vi "Interlock View.vi"(11 "Model in":refnum<class "Model.lvclass">) -> ()   [LabVIEW 2016, in "M1M3SupportEUI_Views.lvlib"]
uses:
  M1M3SupportEUI_Views.lvlib
  Model/Model.lvclass
  M1M3 Support Events/M1M3 Support Events.lvclass/M1M3 Support Events.ctl
  M1M3 Support Events/M1M3 Support Events.lvclass
panel:
  out "GIS Heartbeat Lost":string
  out "TMA Motion Stop":string
  out "Air Supply":string
  out "Thermal Equipment":string
  out "HB Output":string
  out "HB Command":string
  out "Aux Power":string
  out "Heartbeat State":string
  out "AnyWarning":string
  out "Interlock Status Time Stamp":timestamp
  out "Interlock Warning Time Stamp":timestamp
  # "Interlock Event Data"
  # "Warnings"
  # "Status"
  # "Heartbeat Commanded State"
  # "Any Warning"
  # "Heartbeat Output State"
  # "Heartbeat State Output Mismatch"
  # "Critical Fault State Output Mismatch"
  # "Thermal Equipment Off"
  # "Air Supply Off"
  # "TMA Motion Stop"
  # "GIS Heartbeat Lost"
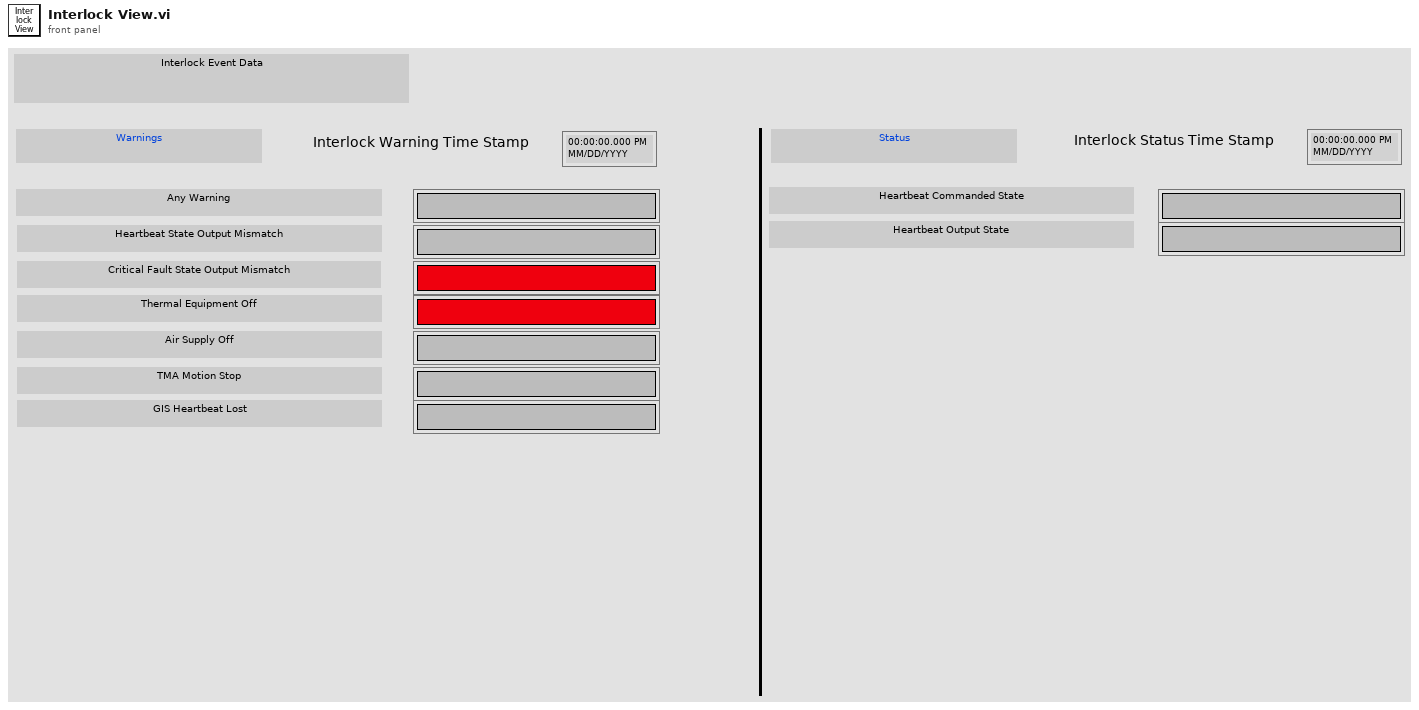
[diagram p1: front panel]
types:
  T1 = typedef "M1M3SupportEUI_TypeDefs.lvlib/M1M3 Support Events.ctl" = cluster{"Inclinometer  Data":refnum<user-event>, "IMS Data":refnum<user-event>, "SAL Connected":refnum<user-event>, "Accelerometer Data":refnum<user-event>, "OuterLoop Data":refnum<user-event>, "ErrorCode Event":refnum<user-event>, "InterlockStatus Event":refnum<user-event>, "InterlockWarning Event":refnum<user-event>, "Gyro Data":refnum<user-event>, "HP Actuator Info Event":refnum<user-event>, " FA Info Event":refnum<user-event>, "HP Monitor Info Event":refnum<user-event>, "FA Data":refnum<user-event>, "HP Actuator data":refnum<user-event>, "HP Monitor data":refnum<user-event>, "Air Supply Status Event":refnum<user-event>, "Air Supply Warning Event":refnum<user-event>, "Power Data":refnum<user-event>, "PID Data":refnum<user-event>, "PID Info Event":refnum<user-event>, "Power Status Event":refnum<user-event>, "Power Supply Status Event":refnum<user-event>, "Power Warning Event":refnum<user-event>, "Summary State Event":refnum<user-event>, "Detailed State Event":refnum<user-event>, "FA Force Warning Event":refnum<user-event>, "FA Warning Event":refnum<user-event>, "FA State Event":refnum<user-event>, "Applied AberrationForces Event":refnum<user-event>, "Applied Acceleration Forcces Event":refnum<user-event>, "Applied Azimuth Forces Event":refnum<user-event>, "Applied Active Optic Forces Event":refnum<user-event>, "Applied Balance Forces Event":refnum<user-event>, "Applied Cylinder Forces Event":refnum<user-event>, "Applied Elevation Forces Event":refnum<user-event>, "Applied Forces Event":refnum<user-event>, "Applied Offset Forces Event":refnum<user-event>, "Applied Static Forces Event":refnum<user-event>, "Applied Thermal Forces Event":refnum<user-event>, "Applied Velocity Forces Event":refnum<user-event>, "Rejected Aberration Force Event":refnum<user-event>, "Rejected Acceleration Forces Event":refnum<user-event>, "Rejected Active Optic Forces Event":refnum<user-event>, "Rejected Azimuth Forces Event":refnum<user-event>, "Rejected Balance Forces Event":refnum<user-event>, "Rejected Cylinder Forces Event":refnum<user-event>, "Rejected Elevation Forces Event":refnum<user-event>, "Rejected Forces Event":refnum<user-event>, "Rejected Offset Forces Event":refnum<user-event>, "Rejected Static Forces Event":refnum<user-event>, "Rejected Thermal Forces Event":refnum<user-event>, "Rejected Velocity Forces Event":refnum<user-event>, "Command Rejection Event":refnum<user-event>, "Setting Verions Event":refnum<user-event>, "Settings Applied Event":refnum<user-event>}
  T2 = enum16{"", "DetailedState_DetailedStates_DisabledState", "DetailedState_DetailedStates_EnabledState", "DetailedState_DetailedStates_FaultState", "DetailedState_DetailedStates_OfflineState", "DetailedState_DetailedStates_StandbyState", "DetailedState_DetailedStates_ParkedState", "DetailedState_DetailedStates_RaisingState", "DetailedState_DetailedStates_ActiveState", "DetailedState_DetailedStates_LoweringState", "DetailedState_DetailedStates_EngineeringState", "DetailedState_DetailedStates_ParkedEngineeringState", "DetailedState_DetailedStates_RaisingEngineeringState", "DetailedState_DetailedStates_ActiveEngineeringState", "DetailedState_DetailedStates_LoweringEngineeringState", "DetailedState_DetailedStates_LoweringFaultState", "DetailedState_DetailedStates_ProfileHardpointCorrectionState"}
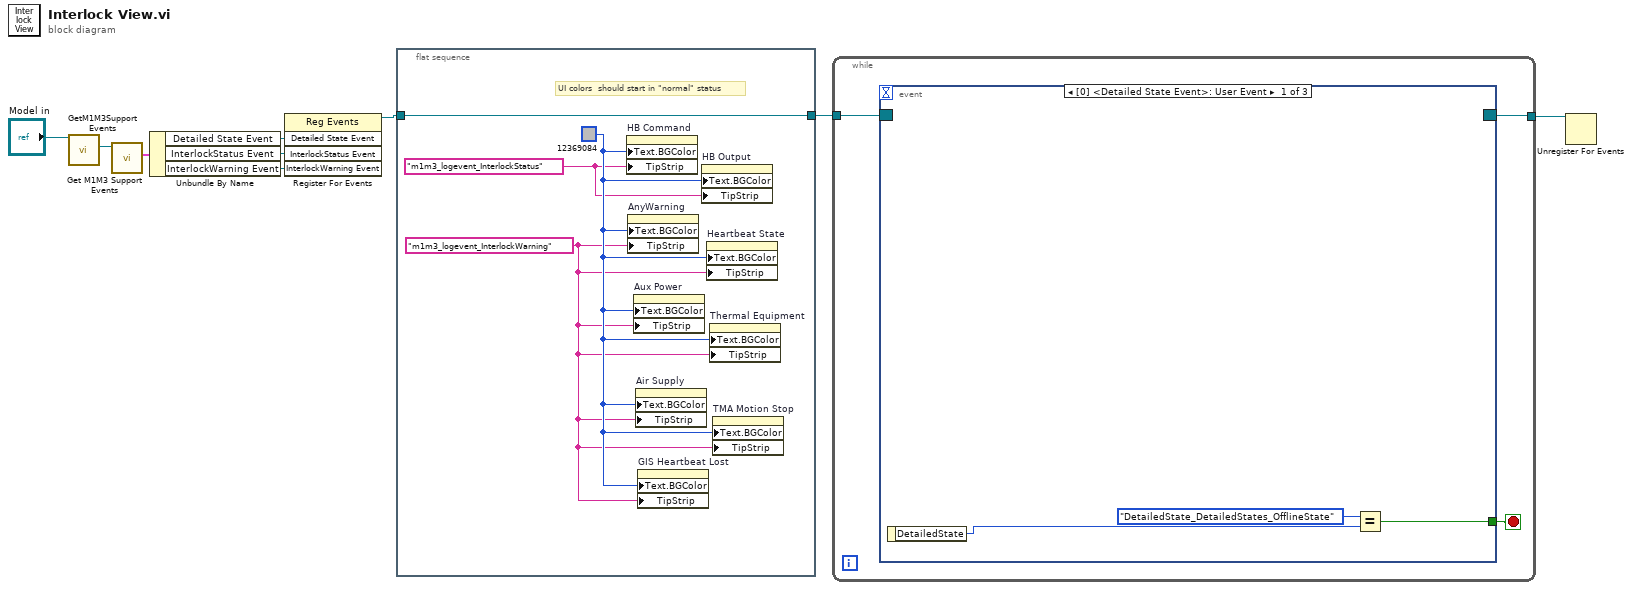
[diagram p0: block diagram]
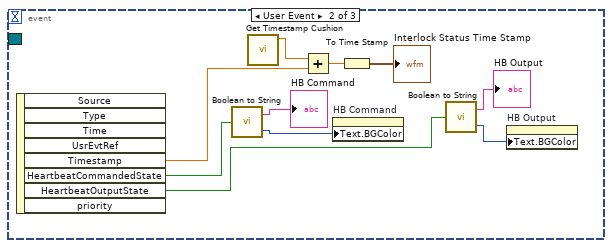
[diagram p2: hidden frame]
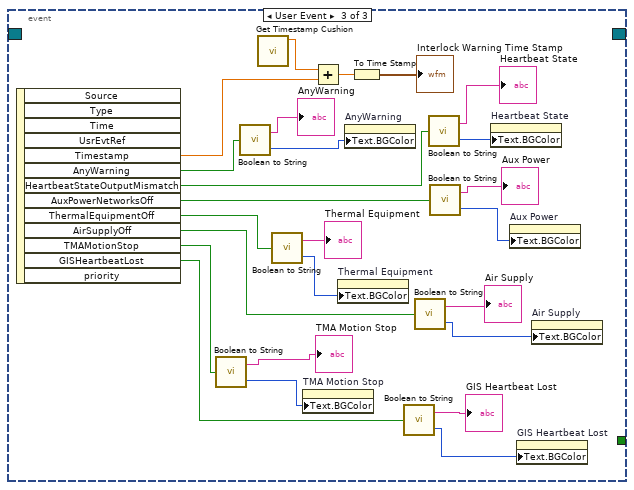
[diagram p3: hidden frame]
diagram:
  n1 = call "GetM1M3SupportEvents.vi"("Model in"="Model in") -> ("M1M3 Support Events out"=w5:refnum<class "M1M3 Support Events.lvclass">)  [unwired: 8 in, 2 out]
  n2 = call "Get M1M3 Support Events.vi"("M1M3 Support Events in"=w5) -> ("M1M3 Support Events"=w6:T1)  [unwired: 9 in, 1 out]
  n3 = Unbundle By Name(w6) -> ("Detailed State Event"=w7:refnum<user-event>, "InterlockStatus Event"=w8:refnum<user-event>, "InterlockWarning Event"=w9:refnum<user-event>)
  n4 = register-events(w7, w8, w9) -> (reference out=w2:refnum<event-registration>)  [unwired: 2 in, 1 out]
  n5 = flat-sequence {
    tunnel: w2 -> [w13]
    tunnel: [w13] -> w1
    frame #0 {
      w10 = "m1m3_logevent_InterlockWarning" ("Tip Strip")
      w11 = "m1m3_logevent_InterlockStatus" ("Tip Strip")
      w12 = u32 12369084
      # "UI colors  should start in \"normal\" status"
      n6 = property on="HB Command" class="Str"("Text.BGColor"=w12, "TipStrip"=w11) -> ()  [unwired: 2 in, 2 out]
      n7 = property on="AnyWarning" class="Str"("Text.BGColor"=w12, "TipStrip"=w10) -> ()  [unwired: 2 in, 2 out]
      n8 = property on="Aux Power" class="Str"("Text.BGColor"=w12, "TipStrip"=w10) -> ()  [unwired: 2 in, 2 out]
      n9 = property on="Air Supply" class="Str"("Text.BGColor"=w12, "TipStrip"=w10) -> ()  [unwired: 2 in, 2 out]
      n10 = property on="GIS Heartbeat Lost" class="Str"("Text.BGColor"=w12, "TipStrip"=w10) -> ()  [unwired: 2 in, 2 out]
      n11 = property on="HB Output" class="Str"("Text.BGColor"=w12, "TipStrip"=w11) -> ()  [unwired: 2 in, 2 out]
      n12 = property on="Heartbeat State" class="Str"("Text.BGColor"=w12, "TipStrip"=w10) -> ()  [unwired: 2 in, 2 out]
      n13 = property on="Thermal Equipment" class="Str"("Text.BGColor"=w12, "TipStrip"=w10) -> ()  [unwired: 2 in, 2 out]
      n14 = property on="TMA Motion Stop" class="Str"("Text.BGColor"=w12, "TipStrip"=w10) -> ()  [unwired: 2 in, 2 out]
    }
  }
  n15 = while {
    tunnel: w1 -> [w16]
    tunnel: [w15] -> w3
    stop <- w14 stop-if-true
    n16 = event shown="[0] <Detailed State Event>: User Event" {
      selector: w16 -> [_ _ _]
      dyn-events: [_ _ _] -> w15
      timeout: _ -> [_ _ _]
      tunnel: [w19 _ _] -> w14
      event User Event {
        n17 = event-data() -> ("DetailedState"=w18:T2)  [unwired: 1 in]
        n18 = Equal?(x=T2."DetailedState_DetailedStates_OfflineState", y=w18) -> (x = y?=w19:bool)
      }
      event User Event {
        n19 = event-data() -> ("Timestamp"=w27:dbl, "HeartbeatCommandedState"=w25:bool, "HeartbeatOutputState"=w22:bool)  [unwired: 1 in, 5 out]
        n20 = call "Boolean to String.vi"("BooleanValue"=w25) -> ("StringForm"=→"HB Command":string, "BackgroundColor"=w23:u32)
        n21 = call "Get Timestamp Cushion.vi"() -> ("TimestampCushion"=w29:dbl)  [unwired: 11 in]
        n22 = Add(x=w29, y=w27) -> (x+y=w28:dbl)
        n23 = property on="HB Command" class="Str"("Text.BGColor"=w23) -> ()  [unwired: 2 in, 2 out]
        n24 = To Time Stamp(1:w28) -> (0:→"Interlock Status Time Stamp":timestamp)
        n25 = call "Boolean to String.vi"("BooleanValue"=w22) -> ("StringForm"=→"HB Output":string, "BackgroundColor"=w20:u32)
        n26 = property on="HB Output" class="Str"("Text.BGColor"=w20) -> ()  [unwired: 2 in, 2 out]
      }
      event User Event {
        n27 = event-data() -> ("Timestamp"=w52:dbl, "AnyWarning"=w50:bool, "HeartbeatStateOutputMismatch"=w47:bool, "AuxPowerNetworksOff"=w44:bool, "ThermalEquipmentOff"=w39:bool, "AirSupplyOff"=w38:bool, "TMAMotionStop"=w35:bool, "GISHeartbeatLost"=w32:bool)  [unwired: 1 in, 5 out]
        n28 = call "Boolean to String.vi"("BooleanValue"=w35) -> ("StringForm"=→"TMA Motion Stop":string, "BackgroundColor"=w33:u32)
        n29 = call "Boolean to String.vi"("BooleanValue"=w50) -> ("StringForm"=→"AnyWarning":string, "BackgroundColor"=w48:u32)
        n30 = call "Get Timestamp Cushion.vi"() -> ("TimestampCushion"=w54:dbl)  [unwired: 11 in]
        n31 = call "Boolean to String.vi"("BooleanValue"=w39) -> ("StringForm"=→"Thermal Equipment":string, "BackgroundColor"=w40:u32)
        n32 = property on="TMA Motion Stop" class="Str"("Text.BGColor"=w33) -> ()  [unwired: 2 in, 2 out]
        n33 = Add(x=w54, y=w52) -> (x+y=w53:dbl)
        n34 = property on="Thermal Equipment" class="Str"("Text.BGColor"=w40) -> ()  [unwired: 2 in, 2 out]
        n35 = property on="AnyWarning" class="Str"("Text.BGColor"=w48) -> ()  [unwired: 2 in, 2 out]
        n36 = To Time Stamp(1:w53) -> (0:→"Interlock Warning Time Stamp":timestamp)
        n37 = call "Boolean to String.vi"("BooleanValue"=w32) -> ("StringForm"=→"GIS Heartbeat Lost":string, "BackgroundColor"=w30:u32)
        n38 = call "Boolean to String.vi"("BooleanValue"=w38) -> ("StringForm"=→"Air Supply":string, "BackgroundColor"=w36:u32)
        n39 = call "Boolean to String.vi"("BooleanValue"=w47) -> ("StringForm"=→"Heartbeat State":string, "BackgroundColor"=w45:u32)
        n40 = call "Boolean to String.vi"("BooleanValue"=w44) -> ("StringForm"=→"Aux Power":string, "BackgroundColor"=w42:u32)
        n41 = property on="Heartbeat State" class="Str"("Text.BGColor"=w45) -> ()  [unwired: 2 in, 2 out]
        n42 = property on="Aux Power" class="Str"("Text.BGColor"=w42) -> ()  [unwired: 2 in, 2 out]
        n43 = property on="GIS Heartbeat Lost" class="Str"("Text.BGColor"=w30) -> ()  [unwired: 2 in, 2 out]
        n44 = property on="Air Supply" class="Str"("Text.BGColor"=w36) -> ()  [unwired: 2 in, 2 out]
      }
    }
  }
  n45 = Unregister For Events(event registration refnum=w3) -> ()  [unwired: 1 in, 1 out]
